vi "Get Timestamp Reference.vi"(8 "error in":errorcluster, 11 "label ref in":T1 format="%.0x") -> (0 "error out":errorcluster, 2 "timestamp channel reference":T1 format="%.0x", 3 "label ref out":T1 format="%.0x", 4 "timestamp channel found?":bool)   [LabVIEW 2020, in "ARINC 429 Scripting.lvlib"]
uses:
  ARINC 429 Scripting.lvlib
  <vilib>/NI VeriStand/Custom Device API/Custom Device Item Ref.ctl
  Constants.vi
  <vilib>/NI VeriStand/Custom Device Tools/Custom Device Utility Library/NI VeriStand - Search for Item by GUID.vi
  <vilib>/NI VeriStand/Custom Device Tools/Custom Device Utility Library/Custom Device Utility Library.lvlib
  Ballard ARINC 429 Scripting.lvlib
  <vilib>/NI VeriStand/Custom Device API/Custom Device API.lvlib
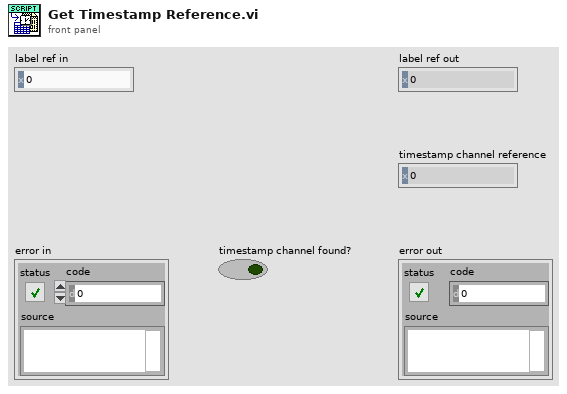
[diagram p1: front panel]
types:
  T1 = typedef "Custom Device API.lvlib/Custom Device Item Ref.ctl" = u64
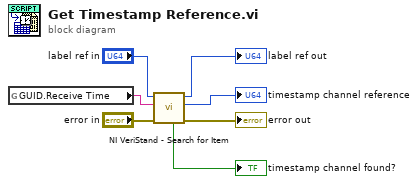
[diagram p0: block diagram]
diagram:
  n1 = global read "Constants.vi" "GUID.Receive Time"() -> (w7:string)
  n2 = call-poly <vilib>:"NI VeriStand - Search for Item.vi"("error in"="error in", "Item GUID"=w7, "Section Ref in"="label ref in") -> ("error out"=→"error out":errorcluster, "Item Ref"=→"timestamp channel reference":T1, "Section Ref out"=→"label ref out":T1, "Found"=→"timestamp channel found?":bool)  [unwired: 5 in]
